vi "公式读取.vi"(8 "Error in":errorcluster caption="Error in (no error)", 10 "量程选择":enum16{"低量程", "高量程", "0-2量程"}(ring), 11 "测量模式(公式)":u16(ring)=1 items=["水样测试"=1, "标样核查"=2, "零点核查"=3, "跨度核查"=4, "空白测试"=5, "平行样"=6, "加标回收"=7]) -> (0 "error out":errorcluster, 3 "方程系数":cluster{"K":dbl, "b":dbl, "X^2":dbl} {"X^2" format="%#.6g"; "b" format="%#.6g"; "K" format="%#.6g"})   [LabVIEW 2016]
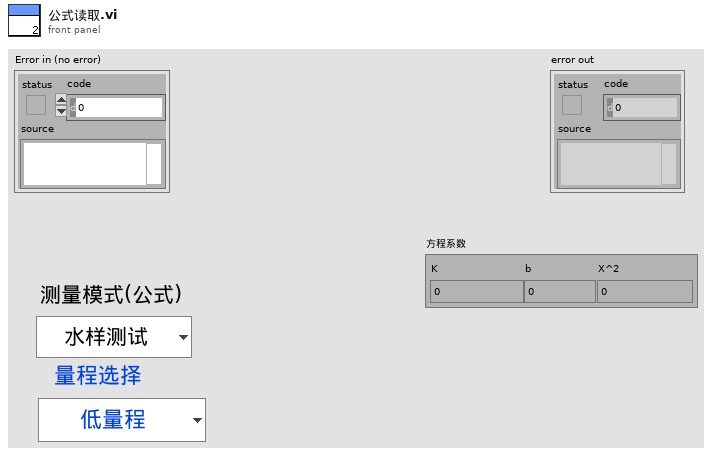
[diagram p1: front panel]
types:
  T1 = cluster{"数组 2[0]":sgl, "数组 2[1]":sgl, "数组 2[2]":sgl, "数组 2[3]":sgl, "数组 2[4]":sgl, "数组 2[5]":sgl, "数组 2[6]":sgl, "数组 2[7]":sgl, "数组 2[8]":sgl, "数组 2[9]":sgl, "数组 2[10]":sgl, "数组 2[11]":sgl, "数组 2[12]":sgl, "数组 2[13]":sgl, "数组 2[14]":sgl, "数组 2[15]":sgl, "数组 2[16]":sgl, "数组 2[17]":sgl, "数组 2[18]":sgl, "数组 2[19]":sgl, "数组 2[20]":sgl, "数组 2[21]":sgl, "数组 2[22]":sgl, "数组 2[23]":sgl, "数组 2[24]":sgl, "数组 2[25]":sgl, "数组 2[26]":sgl, "数组 2[27]":sgl, "数组 2[28]":sgl, "数组 2[29]":sgl, "数组 2[30]":sgl, "数组 2[31]":sgl, "数组 2[32]":sgl, "数组 2[33]":sgl, "数组 2[34]":sgl, "数组 2[35]":sgl, "数组 2[36]":sgl, "数组 2[37]":sgl, "数组 2[38]":sgl, "数组 2[39]":sgl, "数组 2[40]":sgl, "数组 2[41]":sgl}
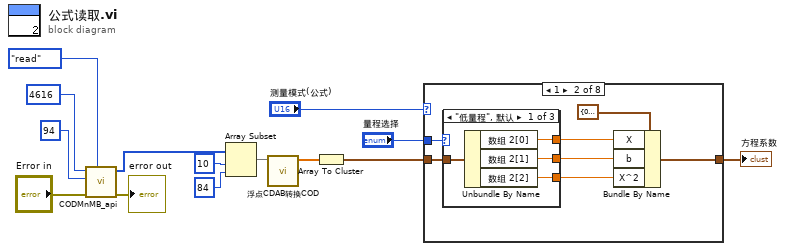
[diagram p0: block diagram]
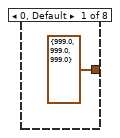
[diagram p2: hidden frame]
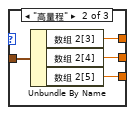
[diagram p3: hidden frame]
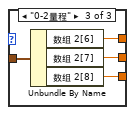
[diagram p4: hidden frame]
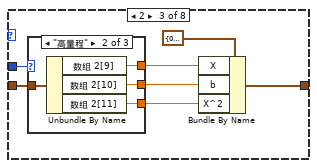
[diagram p5: hidden frame]
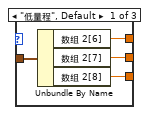
[diagram p6: hidden frame]
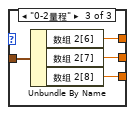
[diagram p7: hidden frame]
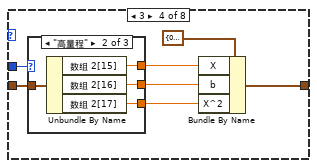
[diagram p8: hidden frame]
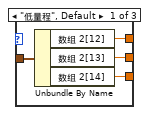
[diagram p9: hidden frame]
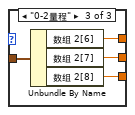
[diagram p10: hidden frame]
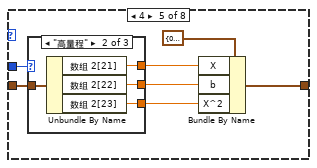
[diagram p11: hidden frame]
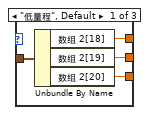
[diagram p12: hidden frame]
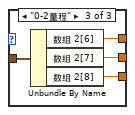
[diagram p13: hidden frame]
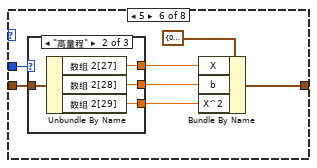
[diagram p14: hidden frame]
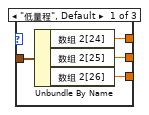
[diagram p15: hidden frame]
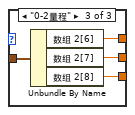
[diagram p16: hidden frame]
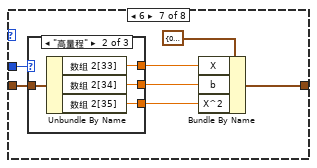
[diagram p17: hidden frame]
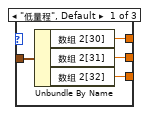
[diagram p18: hidden frame]
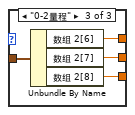
[diagram p19: hidden frame]
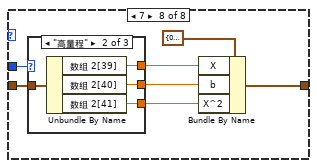
[diagram p20: hidden frame]
diagram:
  n1 = call "CODMnMB_api.vi"("STEP"=enum16{"open", "read", "write", "close"}."read", "Error in"="Error in", "quantity"=u16 94 ("number of holding registers"), "starting address"=u16 4616) -> ("error out"=→"error out":errorcluster, "Registers"=w5:u16[])  [unwired: 5 in, 1 out]
  n2 = Array Subset(array=w5, index=10 ("索引"), length=84 ("长度")) -> (w8:u16[])
  n3 = call "浮点CDAB转换COD.vi"("数组"=w8) -> ("数组 2"=w9:sgl[])  [unwired: 10 in]
  n4 = Array To Cluster(array=w9) -> (cluster=w4:T1)
  n5 = case shown="1" "测量模式(公式)" {
    tunnel: [cluster{"X":dbl, "b":dbl, "X^2":dbl} {"X"=999.0, "b"=999.0, "X^2"=999.0} ("方程系数") w18 w37 w56 w75 w94 w113 w132] -> w2
    tunnel: w4 -> [_ w17 w36 w55 w74 w93 w112 w131]
    tunnel: "量程选择" -> [_ w16 w35 w54 w73 w92 w111 w130]
    frame 0, Default {
    }
    frame 1 {
      n6 = case shown="\"低量程\", 默认" w16 {
        tunnel: w17 -> [w26 w30 w34]
        tunnel: [w25 w29 w33] -> w22
        tunnel: [w24 w28 w32] -> w21
        tunnel: [w23 w27 w31] -> w20
        frame "低量程", Default {
          n7 = Unbundle By Name(w26) -> ("数组 2[0]"=w25:sgl, "数组 2[1]"=w24:sgl, "数组 2[2]"=w23:sgl)
        }
        frame "高量程" {
          n8 = Unbundle By Name(w30) -> ("数组 2[3]"=w29:sgl, "数组 2[4]"=w28:sgl, "数组 2[5]"=w27:sgl)
        }
        frame "0-2量程" {
          n9 = Unbundle By Name(w34) -> ("数组 2[6]"=w33:sgl, "数组 2[7]"=w32:sgl, "数组 2[8]"=w31:sgl)
        }
      }
      n10 = Bundle By Name(cluster=cluster{"X":dbl, "b":dbl, "X^2":dbl} {"X"=0.0, "b"=0.0, "X^2"=0.0} ("方程系数"), "X"=w22, "b"=w21, "X^2"=w20) -> (w18:cluster{"X":dbl, "b":dbl, "X^2":dbl})
    }
    frame 2 {
      n11 = case shown="\"高量程\"" w35 {
        tunnel: w36 -> [w45 w49 w53]
        tunnel: [w44 w48 w52] -> w41
        tunnel: [w43 w47 w51] -> w40
        tunnel: [w42 w46 w50] -> w39
        frame "低量程", Default {
          n12 = Unbundle By Name(w45) -> ("数组 2[6]"=w44:sgl, "数组 2[7]"=w43:sgl, "数组 2[8]"=w42:sgl)
        }
        frame "高量程" {
          n13 = Unbundle By Name(w49) -> ("数组 2[9]"=w48:sgl, "数组 2[10]"=w47:sgl, "数组 2[11]"=w46:sgl)
        }
        frame "0-2量程" {
          n14 = Unbundle By Name(w53) -> ("数组 2[6]"=w52:sgl, "数组 2[7]"=w51:sgl, "数组 2[8]"=w50:sgl)
        }
      }
      n15 = Bundle By Name(cluster=cluster{"X":dbl, "b":dbl, "X^2":dbl} {"X"=0.0, "b"=0.0, "X^2"=0.0} ("方程系数"), "X"=w41, "b"=w40, "X^2"=w39) -> (w37:cluster{"X":dbl, "b":dbl, "X^2":dbl})
    }
    frame 3 {
      n16 = case shown="\"高量程\"" w54 {
        tunnel: w55 -> [w64 w68 w72]
        tunnel: [w63 w67 w71] -> w60
        tunnel: [w62 w66 w70] -> w59
        tunnel: [w61 w65 w69] -> w58
        frame "低量程", Default {
          n17 = Unbundle By Name(w64) -> ("数组 2[12]"=w63:sgl, "数组 2[13]"=w62:sgl, "数组 2[14]"=w61:sgl)
        }
        frame "高量程" {
          n18 = Unbundle By Name(w68) -> ("数组 2[15]"=w67:sgl, "数组 2[16]"=w66:sgl, "数组 2[17]"=w65:sgl)
        }
        frame "0-2量程" {
          n19 = Unbundle By Name(w72) -> ("数组 2[6]"=w71:sgl, "数组 2[7]"=w70:sgl, "数组 2[8]"=w69:sgl)
        }
      }
      n20 = Bundle By Name(cluster=cluster{"X":dbl, "b":dbl, "X^2":dbl} {"X"=0.0, "b"=0.0, "X^2"=0.0} ("方程系数"), "X"=w60, "b"=w59, "X^2"=w58) -> (w56:cluster{"X":dbl, "b":dbl, "X^2":dbl})
    }
    frame 4 {
      n21 = case shown="\"高量程\"" w73 {
        tunnel: w74 -> [w83 w87 w91]
        tunnel: [w82 w86 w90] -> w79
        tunnel: [w81 w85 w89] -> w78
        tunnel: [w80 w84 w88] -> w77
        frame "低量程", Default {
          n22 = Unbundle By Name(w83) -> ("数组 2[18]"=w82:sgl, "数组 2[19]"=w81:sgl, "数组 2[20]"=w80:sgl)
        }
        frame "高量程" {
          n23 = Unbundle By Name(w87) -> ("数组 2[21]"=w86:sgl, "数组 2[22]"=w85:sgl, "数组 2[23]"=w84:sgl)
        }
        frame "0-2量程" {
          n24 = Unbundle By Name(w91) -> ("数组 2[6]"=w90:sgl, "数组 2[7]"=w89:sgl, "数组 2[8]"=w88:sgl)
        }
      }
      n25 = Bundle By Name(cluster=cluster{"X":dbl, "b":dbl, "X^2":dbl} {"X"=0.0, "b"=0.0, "X^2"=0.0} ("方程系数"), "X"=w79, "b"=w78, "X^2"=w77) -> (w75:cluster{"X":dbl, "b":dbl, "X^2":dbl})
    }
    frame 5 {
      n26 = case shown="\"高量程\"" w92 {
        tunnel: w93 -> [w102 w106 w110]
        tunnel: [w101 w105 w109] -> w98
        tunnel: [w100 w104 w108] -> w97
        tunnel: [w99 w103 w107] -> w96
        frame "低量程", Default {
          n27 = Unbundle By Name(w102) -> ("数组 2[24]"=w101:sgl, "数组 2[25]"=w100:sgl, "数组 2[26]"=w99:sgl)
        }
        frame "高量程" {
          n28 = Unbundle By Name(w106) -> ("数组 2[27]"=w105:sgl, "数组 2[28]"=w104:sgl, "数组 2[29]"=w103:sgl)
        }
        frame "0-2量程" {
          n29 = Unbundle By Name(w110) -> ("数组 2[6]"=w109:sgl, "数组 2[7]"=w108:sgl, "数组 2[8]"=w107:sgl)
        }
      }
      n30 = Bundle By Name(cluster=cluster{"X":dbl, "b":dbl, "X^2":dbl} {"X"=0.0, "b"=0.0, "X^2"=0.0} ("方程系数"), "X"=w98, "b"=w97, "X^2"=w96) -> (w94:cluster{"X":dbl, "b":dbl, "X^2":dbl})
    }
    frame 6 {
      n31 = case shown="\"高量程\"" w111 {
        tunnel: w112 -> [w121 w125 w129]
        tunnel: [w120 w124 w128] -> w117
        tunnel: [w119 w123 w127] -> w116
        tunnel: [w118 w122 w126] -> w115
        frame "低量程", Default {
          n32 = Unbundle By Name(w121) -> ("数组 2[30]"=w120:sgl, "数组 2[31]"=w119:sgl, "数组 2[32]"=w118:sgl)
        }
        frame "高量程" {
          n33 = Unbundle By Name(w125) -> ("数组 2[33]"=w124:sgl, "数组 2[34]"=w123:sgl, "数组 2[35]"=w122:sgl)
        }
        frame "0-2量程" {
          n34 = Unbundle By Name(w129) -> ("数组 2[6]"=w128:sgl, "数组 2[7]"=w127:sgl, "数组 2[8]"=w126:sgl)
        }
      }
      n35 = Bundle By Name(cluster=cluster{"X":dbl, "b":dbl, "X^2":dbl} {"X"=0.0, "b"=0.0, "X^2"=0.0} ("方程系数"), "X"=w117, "b"=w116, "X^2"=w115) -> (w113:cluster{"X":dbl, "b":dbl, "X^2":dbl})
    }
    frame 7 {
      n36 = case shown="\"高量程\"" w130 {
        tunnel: w131 -> [w140 w144 w148]
        tunnel: [w139 w143 w147] -> w136
        tunnel: [w138 w142 w146] -> w135
        tunnel: [w137 w141 w145] -> w134
        frame "低量程", Default {
          n37 = Unbundle By Name(w140) -> ("数组 2[36]"=w139:sgl, "数组 2[37]"=w138:sgl, "数组 2[38]"=w137:sgl)
        }
        frame "高量程" {
          n38 = Unbundle By Name(w144) -> ("数组 2[39]"=w143:sgl, "数组 2[40]"=w142:sgl, "数组 2[41]"=w141:sgl)
        }
        frame "0-2量程" {
          n39 = Unbundle By Name(w148) -> ("数组 2[6]"=w147:sgl, "数组 2[7]"=w146:sgl, "数组 2[8]"=w145:sgl)
        }
      }
      n40 = Bundle By Name(cluster=cluster{"X":dbl, "b":dbl, "X^2":dbl} {"X"=0.0, "b"=0.0, "X^2"=0.0} ("方程系数"), "X"=w136, "b"=w135, "X^2"=w134) -> (w132:cluster{"X":dbl, "b":dbl, "X^2":dbl})
    }
  }
  "方程系数" <- w2
